vi "Debug Test.vi"() -> ()   [LabVIEW 2009]
uses:
  Debug Shared/Control Information.ctl
  cRIO/Sensors/Sensor Typedefs/FPGA Main ref.ctl
  cRIO/Sensors/Sensor Typedefs/GPS Data.ctl
  cRIO/Sensors/Sensor Typedefs/SICK Array.ctl
  Remote Control/Motor Command.ctl
  cRIO/Queue Type Def's/Motor State.ctl
  cRIO/Queue Type Def's/Motor Instruction.ctl
  cRIO/Startup VI Support Files/Main State.ctl
  Remote Control/Control Message.ctl
panel:
  out "Control Info.":T1
  out "HB":bool
  in  "Safety Disabled":bool
  in  "Camera  Init Complete":bool
  out "HB":bool
  in  "Control Message":T2
  out "RC/!Run":bool=TRUE
  out "Main State":T4=enum."Remote Control"
  out "MC VISA resource":refnum<visa-resource-name>="ASRL1::INSTR"
  in  "Motors Init Complete":bool=TRUE
  out "Motor Queue":refnum<queue>
  in  "RC Command Buffer":T3
  in  "Motors On?":bool=TRUE
  in  "Sensors Init Complete":bool=TRUE
  in  "SICK Buffer":T5
  in  "Compass Buffer":dbl=181.1
  in  "Compass Init Complete":bool
  in  "SICK Init Complete":bool
  in  "GPS Init Complete":bool
  in  "GPS Buffer":T6
  out "FPGA VI Reference":T7
  in  "Motor Message":string
  out "VFH Queue":refnum<queue>
  out "Communication Queue":refnum<queue>
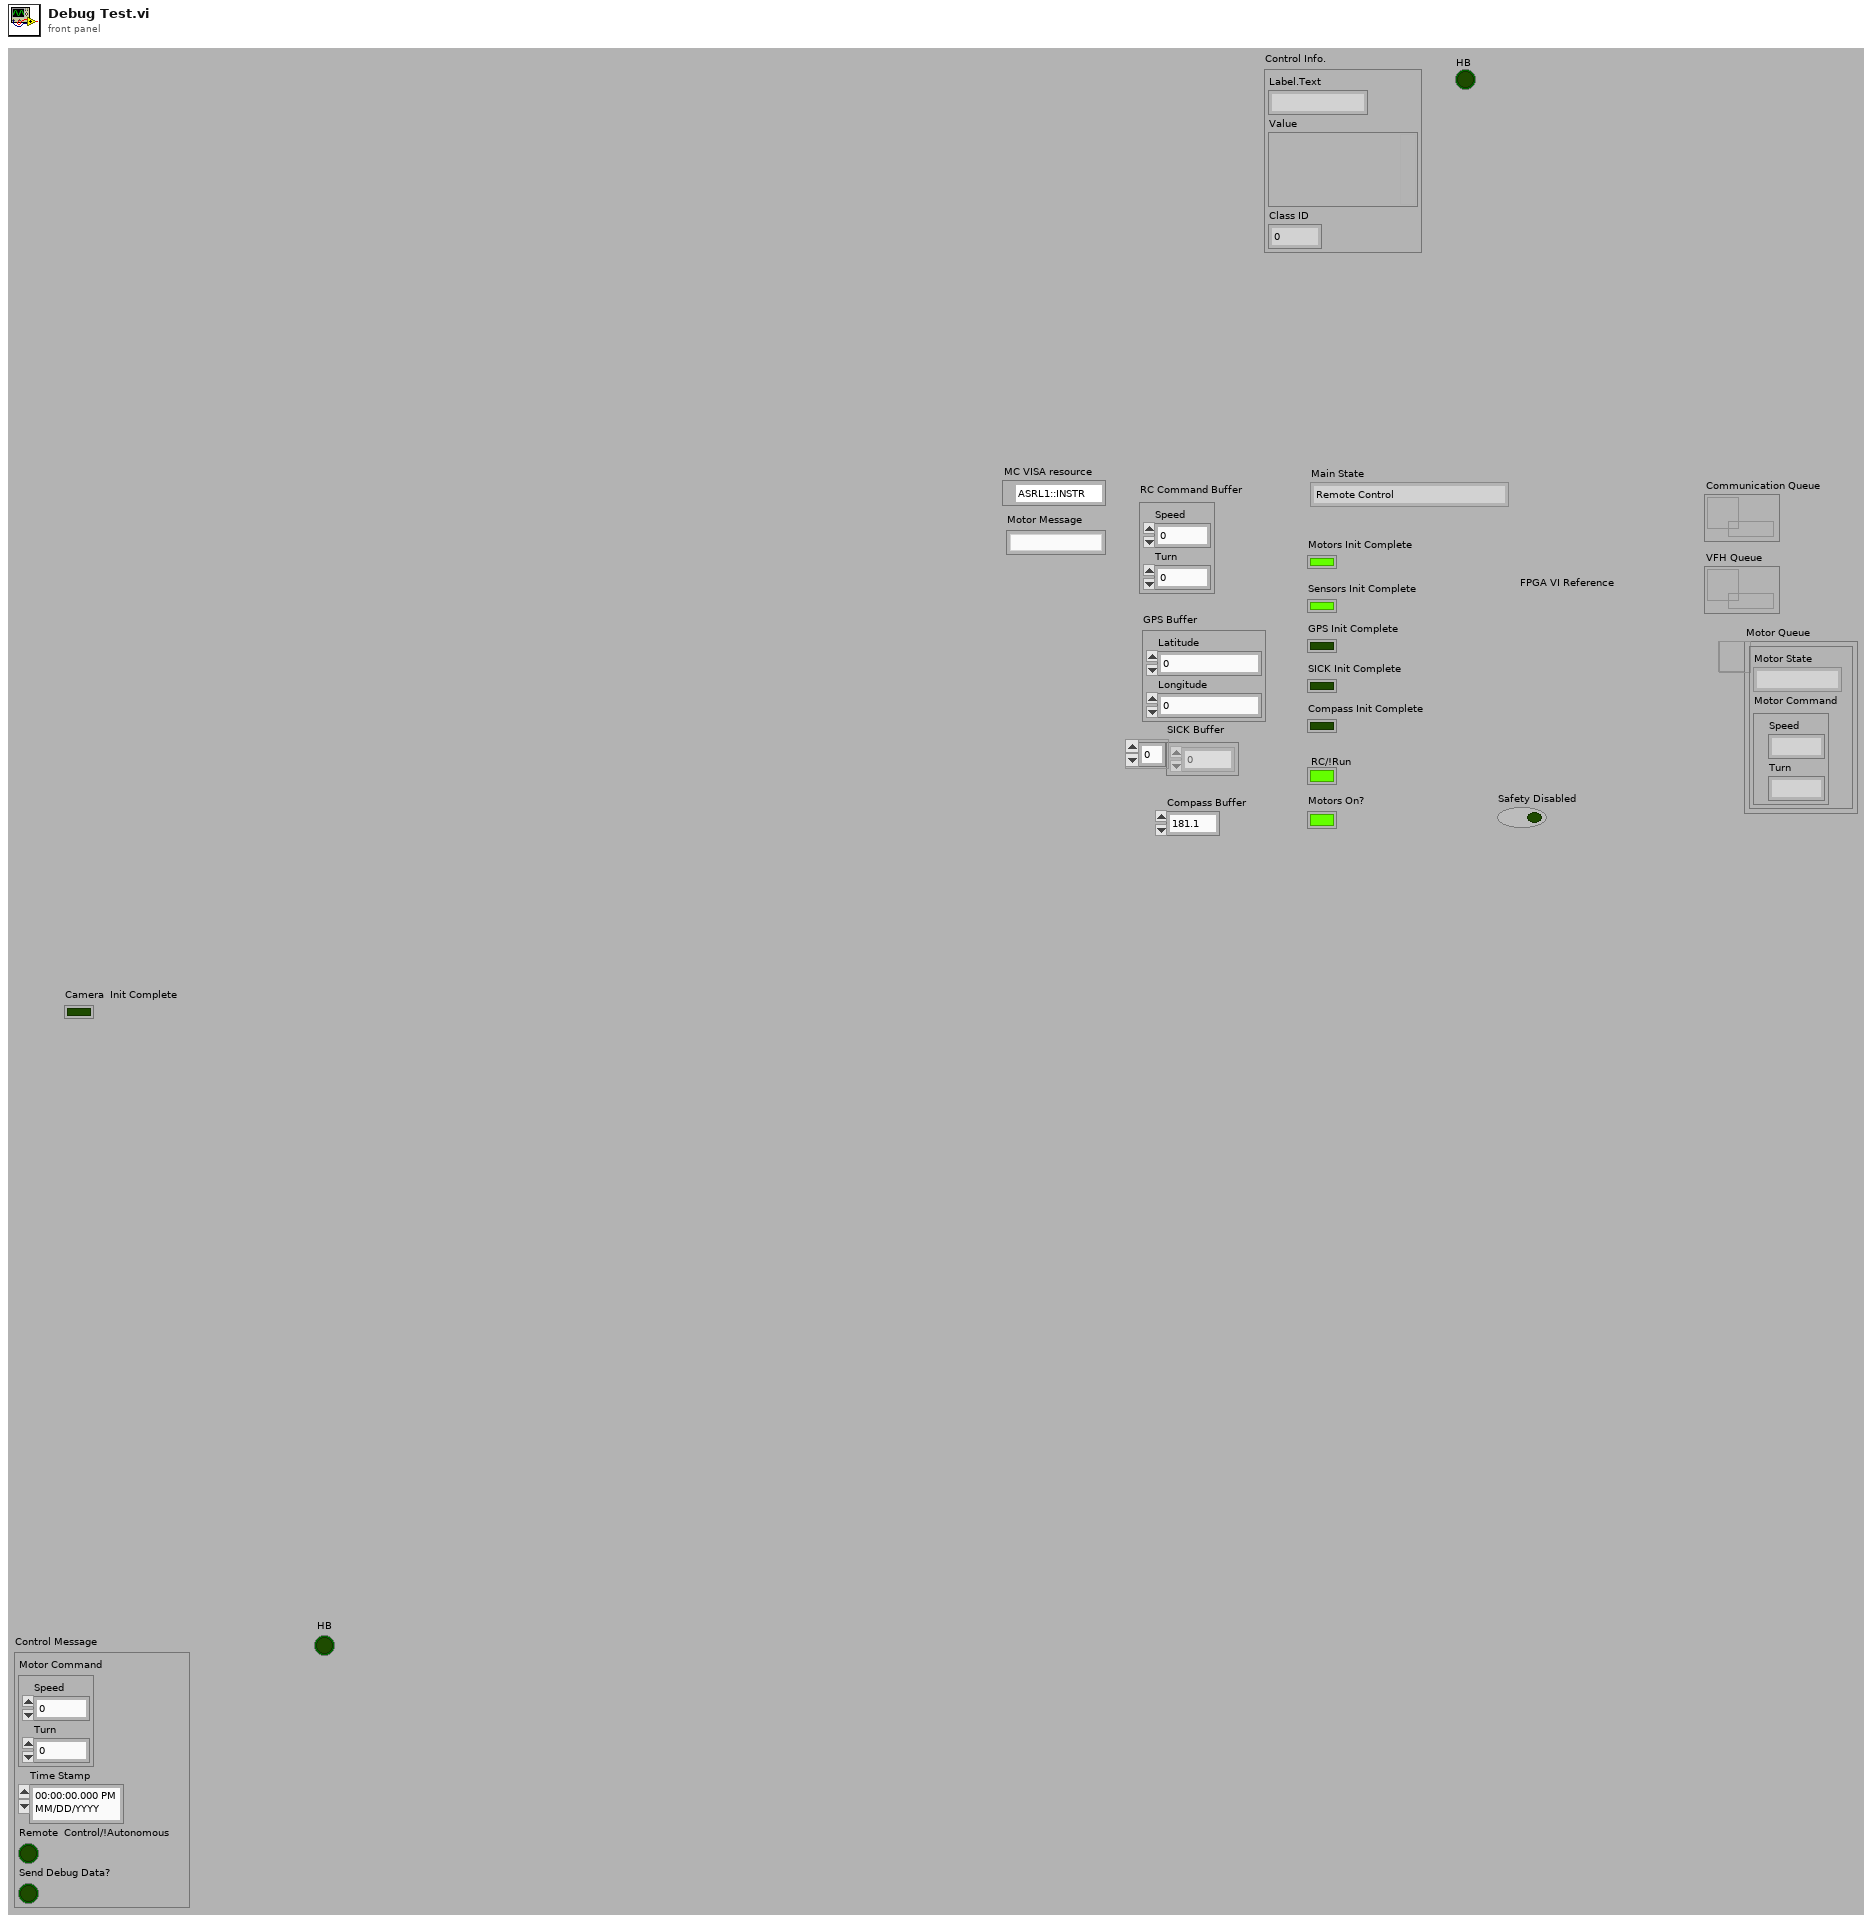
[diagram p1: front panel]
types:
  T1 = typedef "Control Information.ctl" = cluster{"Label.Text":string, "Value":variant, "Class ID":u32}
  T2 = typedef "Control Message.ctl" = cluster{"Motor Command":T3, "Time Stamp":timestamp, "Remote  Control/!Autonomous":bool, "Send Debug Data?":bool}
  T3 = typedef "Motor Command.ctl" = cluster{"Speed":i16, "Turn":i16}
  T4 = typedef "Main State.ctl" = enum16{"Initialize Sensors", "Initialize Motors", "Wait for GO", "Run", "Remote Control", "Stop"}
  T5 = typedef "SICK Array.ctl" = u16[]
  T6 = typedef "GPS Data.ctl" = cluster{"Latitude":dbl, "Longitude":dbl}
  T7 = typedef "FPGA Main ref.ctl" = refnum<k20>
  T8 = typedef "UDP Base.ctl" = cluster{"UDP Session":refnum<k16>, "UDP Socket Params":T9}
  T9 = typedef "UDP Socket Params.ctl" = cluster{"Local Port":u16, "Read Timeout":i32, "Write Timeout":i32}
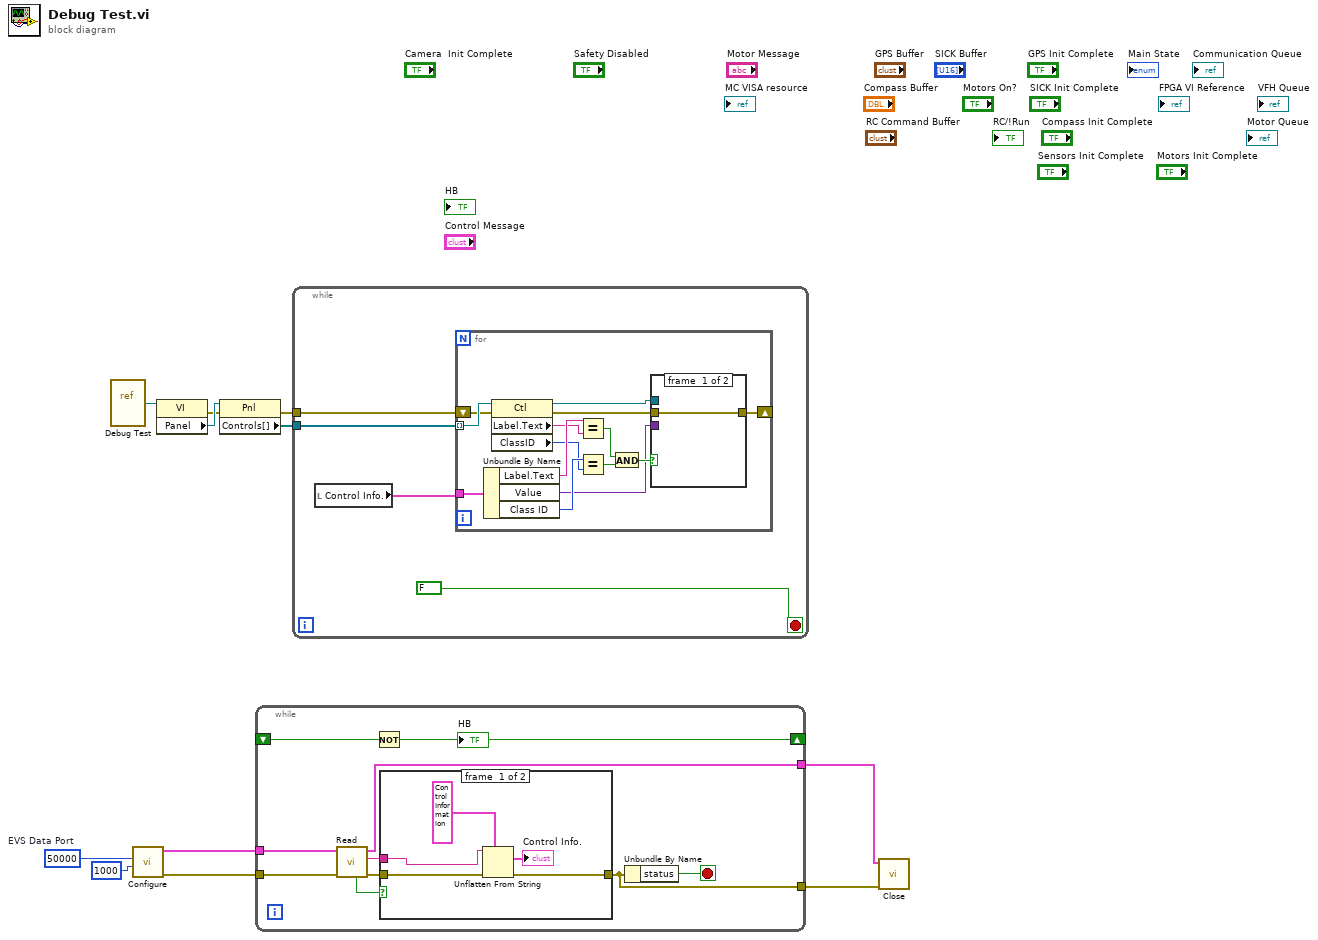
[diagram p0: block diagram]
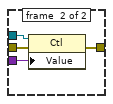
[diagram p3: hidden frame]
diagram:
  w3 = u16 50000  # EVS Data Port
  n1 = vi-ref "Debug Test.vi"() -> (w10:refnum<vi>)
  n2 = call "Configure.vi"("Read Timeout"=1000, "Local Port"=w3) -> ("error out"=w2:errorcluster, "UDP Base out"=w1:T8)  [unwired: 8 in]
  n3 = property class="VI"(reference=w10) -> (error out=w8:errorcluster, "Panel"=w11:refnum<vi>)  [unwired: 1 in, 1 out]
  n4 = property class="Pnl"(reference=w11, error in=w8) -> (error out=w7:errorcluster, "Controls[]"=w9:refnum<vi>[])  [unwired: 1 out]
  n5 = while {
    tunnel: w1 -> [w21]
    tunnel: w2 -> [w20]
    tunnel: [w12] -> w6
    tunnel: [w19] -> w5
    shift-right: [w17] -> _
    shift-left: _ -> [w18]
    stop <- w13 stop-if-true
    n6 = call "Read.vi"("error in (no error)"=w20, "UDP Base in"=w21) -> ("error out"=w16:errorcluster, "Receive Data"=w15:string, "UDP Base out"=w19:T8, "Timeout"=w14:bool)  [unwired: 4 in, 2 out]
    n7 = Not(x=w18) -> (.not. x?=w17:bool)
    "HB" <- w17
    n8 = case shown="False" w14 {
      tunnel: w16 -> [w26 w27]
      tunnel: [w25 w27] -> w12
      tunnel: w15 -> [w24 _]
      frame #0 {
        n9 = Unflatten From String(type=T1 {"Label.Text"="", "Value"=variant, "Class ID"=0} ("Control Information"), binary string=w24, error in (no error)=w26) -> (value=→"Control Info.":T1, error out=w25:errorcluster)  [unwired: 2 in, 1 out]
      }
      frame #1 {
      }
    }
    n10 = Unbundle By Name(w12) -> ("status"=w13:bool)
  }
  n11 = while {
    tunnel: w9 -> [w31]
    tunnel: w7 -> [w30]
    stop <- FALSE ("stop") stop-if-true
    n12 = local read "Control Info."() -> (w28:T1)
    n13 = for {
      tunnel: w28 -> [w45]
      tunnel: w31 -> [w44] mode=indexing
      shift-right: [w33] -> _
      shift-left: w30 -> [w35]
      n14 = Unbundle By Name(w45) -> ("Label.Text"=w43:string, "Value"=w32:variant, "Class ID"=w41:u32)
      n15 = property class="Ctl"(reference=w44, error in=w35) -> (reference out=w36:refnum<vi>, error out=w34:errorcluster, "Label.Text"=w42:string, "ClassID"=w40:u32)
      n16 = Equal?(x=w43, y=w42) -> (x = y?=w38:bool)
      n17 = Equal?(x=w41, y=w40) -> (x = y?=w39:bool)
      n18 = And(x=w38, y=w39) -> (x .and. y?=w37:bool)
      n19 = case shown="True" w37 {
        tunnel: w36 -> [_ w50]
        tunnel: w34 -> [w46 w49]
        tunnel: [w46 w48] -> w33
        tunnel: w32 -> [_ w47]
        frame #0 {
        }
        frame #1 {
          n20 = property class="Ctl"(reference=w50, error in=w49, "Value"=w47) -> (error out=w48:errorcluster)  [unwired: 1 out]
        }
      }
    }
  }
  n21 = call "Close.vi"("error in (no error)"=w6, "Cluster of class private data"=w5) -> ()  [unwired: 9 in, 1 out]
